vi "stackInGrid.vi"(4 "preferredDirection":T1, 5 "verticalSpacing":u16, 6 "elementsInPreferredDirection":i32, 7 "horizontalSpacing":u16, 8 "error in (no error)":errorcluster, 9 "useControlBodyOnly":bool, 11 "refs":refnum<vi>[](array[refnum])) -> (0 "error out":errorcluster, 3 "refs(dup)":refnum<vi>[](array[refnum]))   [LabVIEW 2023, in "TLC_Geometry.lvlib"]
doc: "Stacks the input controls into a structured grid layout.\nArranges the controls using the specified horizontal and vertical spacing. Controls are positioned according to their order in the array.\nThe preferred direction determines whether the grid is filled row-wise (horizontal) or column-wise (vertical).\nThe number of elements in the preferred direction defines the number of columns (if horizontal) or rows (if vertical).\nControl sizes are preserved.\nColumn widths and row heights are determined by the maximum size of the controls within each column or row."
uses:
  TLC_Geometry.lvlib
  direction.ctl
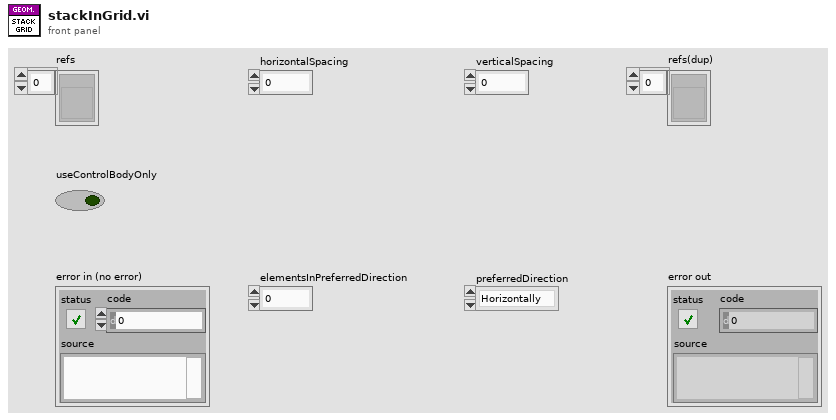
[diagram p1: front panel]
types:
  T1 = typedef "TLC_Geometry.lvlib/direction.ctl" = enum16{"Horizontally", "Vertically"}
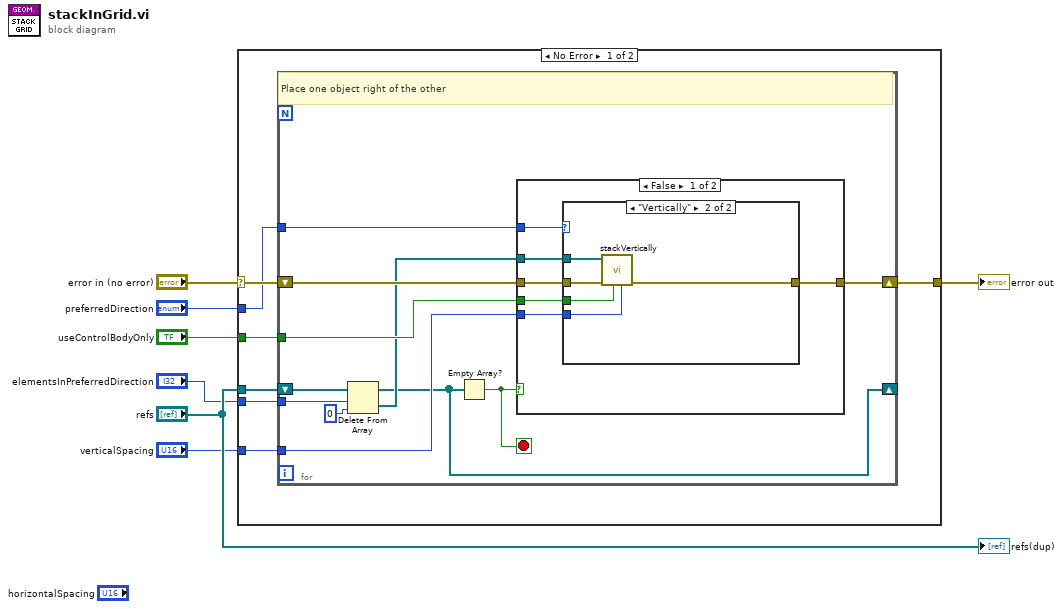
[diagram p0: block diagram]
diagram:
  n1 = case shown="No Error" "error in (no error)" {
    selector: "error in (no error)" -> [w14 w38]
    tunnel: [w13 w38] -> w4
    tunnel: "refs" -> [w9 _]
    tunnel: "useControlBodyOnly" -> [w12 _]
    tunnel: "verticalSpacing" -> [w11 _]
    tunnel: "preferredDirection" -> [w10 _]
    tunnel: "elementsInPreferredDirection" -> [w8 _]
    frame No Error {
      n2 = for {
        shift-right: [w24] -> w13
        shift-left: w14 -> [w25]
        tunnel: w12 -> [w23]
        tunnel: w11 -> [w22]
        tunnel: w10 -> [w21]
        shift-right: [w16] -> _
        shift-left: w9 -> [w20]
        tunnel: w8 -> [w19]
        stop <- w15 stop-if-true
        # "Place one object right of the other"
        n3 = Delete From Array(array=w20, length=w19, index=0) -> (deleted portion=w17:refnum<vi>[], array with subset deleted=w16:refnum<vi>[])
        n4 = Empty Array?(array=w16) -> (empty?=w15:bool)
        n5 = case shown="False" w15 {
          tunnel: w25 -> [w31 _]
          tunnel: [w30 _] -> w24
          tunnel: w23 -> [w29 _]
          tunnel: w22 -> [w28 _]
          tunnel: w21 -> [w27 _]
          tunnel: w17 -> [w26 _]
          frame False {
            n6 = case shown="\"Vertically\"" w27 {
              tunnel: w31 -> [w32 w37]
              tunnel: [w32 w36] -> w30
              tunnel: w29 -> [_ w35]
              tunnel: w28 -> [_ w34]
              tunnel: w26 -> [_ w33]
              frame "Horizontally", Default {
              }
              frame "Vertically" {
                n7 = call "stackVertically.vi"("spacing"=w34, "useControlBodyOnly"=w35, "error in (no error)"=w37, "refs"=w33) -> ("error out"=w36:errorcluster)  [unwired: 6 in, 1 out]
              }
            }
          }
          frame True {
          }
        }
      }
    }
    frame Error {
    }
  }
  "error out" <- w4
  "refs(dup)" <- "refs"
